vi "Test Code Block.vi"() -> ()   [LabVIEW 2014]
uses:
  <vilib>/Aledyne-TSXperts/Arduino Compatible Compiler for LabVIEW/addons/Arduino Extra Functions/Arduino Extra Functions.lvlib
panel:
  out "Error Out":errorcluster
  in  "Error In":errorcluster
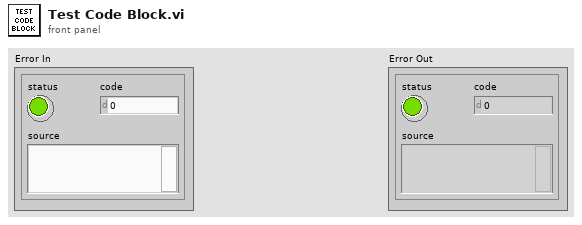
[diagram p1: front panel]
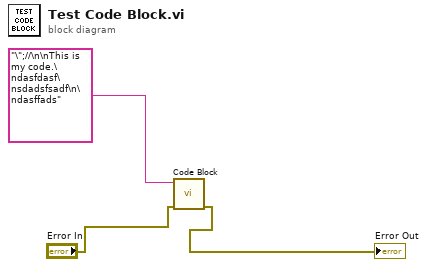
[diagram p0: block diagram]
diagram:
  n1 = call <vilib>:"Code Block.vi"("Error In"="Error In", "Code"="\";//\n\nThis is my code.\ndasfdasf\nsdadsfsadf\n\ndasffads") -> ("Error Out"=→"Error Out":errorcluster)  [unwired: 9 in]
